vi "stoperaseCI.vi"   [LabVIEW 2015]
types:
  T1 = typedef "LVRectTypeDef.ctl" = cluster{"Left":i16, "Top":i16, "Right":i16, "Bottom":i16}
  T2 = cluster{"Xpixels":i32, "Vxminref":dbl, "Vxmaxref":dbl, "P":dbl, "Ypixels":i32, "Vyminref":dbl, "Vymaxref":dbl, "srate":sgl, "sAOxy":i32, "timeout":dbl, "type":string, "date":string, "time":string, "Colormap":u16, "Drawing Mode":u16, "Scanning Mode":u16, "square pixels":bool, "square matrix":bool, "Xpixels Img":i32, "Vx-min Img":dbl, "VX-max Img":dbl, "Ypixels Img":i32, "Vy-min Img":dbl, "Vy-max Img ":dbl, "Angle Img":dbl, "autoshutter":bool, "finite":bool, "cont":bool, "wavdet":bool, "measpoints":i32, "avpp":i32, "bufferAO":i32, "bufferAI":i32, "starttick":u32, "waveform":path, "Vx-ref":dbl, "Vy-ref":dbl, "refreshrate":dbl, "refreshbuffer":i32, "tt_cycles":i32, "motorref":refnum<k7>, "mirrorswitch":refnum<k7>, "sample mode":i32, "maxbufferAI":i32, "srateAODO":sgl, "bin":sgl, "Pel":sgl, "Angle draw":dbl, "srate Img":sgl, "ROIimg_plotbounds":T1, "auto OD":bool, "ODfilt":u16, "aAI":i32[], "aCI":i32[], "aAO":u32[], "aDO":u32[], "refwfsize":dbl, "Lifetime":bool, "Vz-Img":dbl, "Vz-ref":dbl, "Vz-reset":dbl, "AIoverride":bool, "aAS":u32[], "XYZstart":dbl[]}
  T3 = cluster{"CI":refnum<k21>[], "E_CI":errorcluster[]}
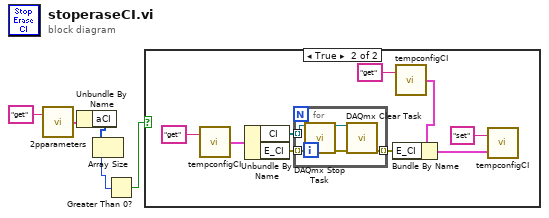
[diagram p0: block diagram]
diagram:
  n1 = call "2pparameters.vi"("command"="get") -> ("params out"=w4:T2)  [unwired: 1 in]
  n2 = Unbundle By Name(w4) -> ("aCI"=w1:i32[])
  n3 = Array Size(array=w1) -> (size(s)=w3:i32)
  n4 = Greater Than 0?(x=w3) -> (x > 0?=w2:bool)
  n5 = case shown="True" w2 {
    frame False {
    }
    frame True {
      n6 = call "tempconfigCI.vi"("command"="get") -> ("Temp Config out"=w13:T3)  [unwired: 1 in]
      n7 = Unbundle By Name(w13) -> ("CI"=w12:refnum<k21>[], "E_CI"=w11:errorcluster[])
      n8 = for {
        tunnel: w12 -> [w17] mode=indexing
        tunnel: w11 -> [w16] mode=indexing
        tunnel: [w15] -> w7 mode=indexing
        n9 = call <vilib>:"DAQmx Stop Task.vi"("task/channels in"=w17, "error in"=w16) -> ("task out"=w18:refnum<k21>, "error out"=w19:errorcluster)  [unwired: 12 in]
        n10 = call <vilib>:"DAQmx Clear Task.vi"("task in"=w18, "error in"=w19) -> ("error out"=w15:errorcluster)  [unwired: 13 in]
      }
      n11 = call "tempconfigCI.vi"("command"="get") -> ("Temp Config out"=w8:T3)  [unwired: 1 in]
      n12 = Bundle By Name(cluster=w8, "E_CI"=w7) -> (w6:T3)
      n13 = call "tempconfigCI.vi"("Temp Config in"=w6, "command"="set") -> ()  [unwired: 1 out]
    }
  }
